vi "Set Temperature.vi"(4 "Channel":i32, 8 "error in (no error)":errorcluster, 9 "Rate (K/min)":dbl, 10 "Temperature (K)":dbl, 11 "instrument.PPMS2 in":refnum<class "instrument.PPMS2.lvclass">) -> (0 "error out":errorcluster, 3 "instrument.PPMS2 out":refnum<class "instrument.PPMS2.lvclass">)   [LabVIEW 2016, in "instrument.PPMS2.lvclass"]
uses:
  instrument.PPMS2.lvclass
  Typedefs/Temperature--PPMS2--cluster.ctl
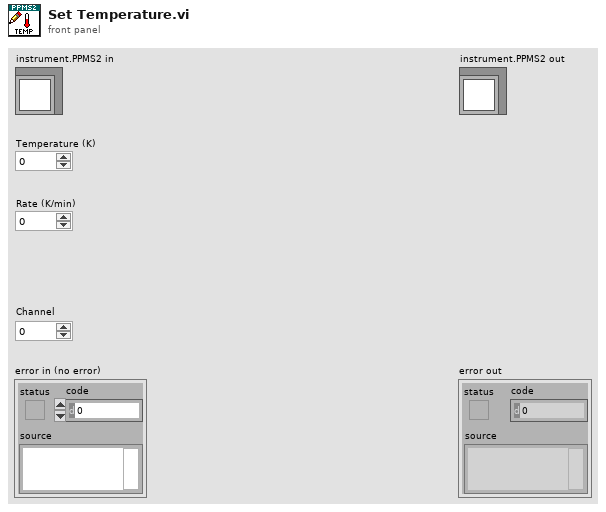
[diagram p1: front panel]
types:
  T1 = typedef "instrument.PPMS2.lvclass/Temperature--PPMS2--cluster.ctl" = cluster{"Temperature (K)":dbl, "Rate (K/min)":dbl}
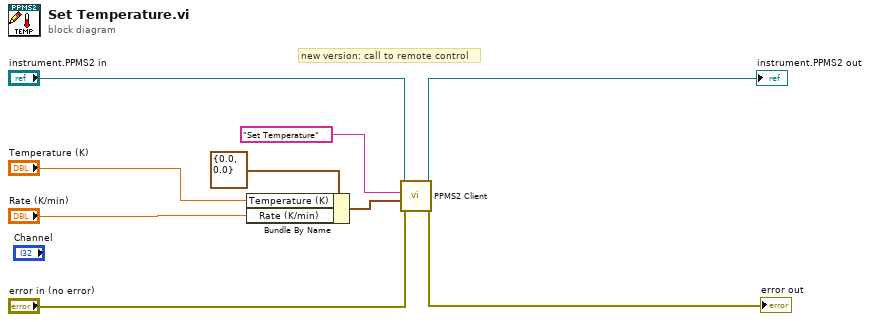
[diagram p0: block diagram]
diagram:
  # "new version: call to remote control"
  n1 = Bundle By Name(cluster=T1 {"Temperature (K)"=0.0, "Rate (K/min)"=0.0} ("output cluster"), "Temperature (K)"="Temperature (K)", "Rate (K/min)"="Rate (K/min)") -> (w2:T1)
  n2 = call "PPMS2 Client.vi"("error in (no error)"="error in (no error)", "Data"=w2, "Command"="Set Temperature", "instrument.PPMS2 in"="instrument.PPMS2 in") -> ("error out"=→"error out":errorcluster, "instrument.PPMS2 out"=→"instrument.PPMS2 out":refnum<class "instrument.PPMS2.lvclass">)  [unwired: 4 in, 2 out]
